vi "GetSetTopSponsorImage.vi"(8 "Which":enum16{"Low", "Mid", "Top"}(ring), 9 "Get/Set":enum16{"Get", "Set"}(ring), 11 "image data":T1) -> (3 "image data out":T1)   [LabVIEW 2013]
uses:
  <vilib>/picture/picture.llb/imagedata.ctl
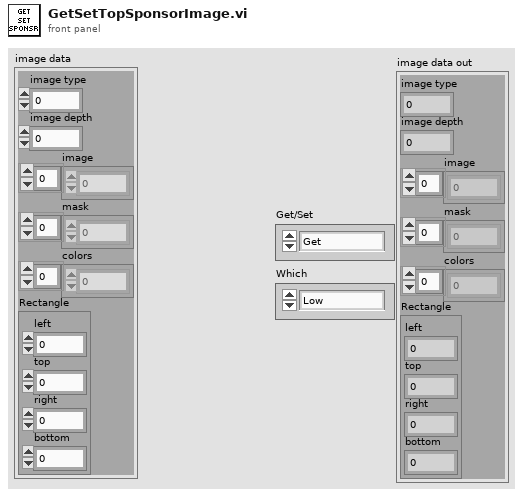
[diagram p1: front panel]
types:
  T1 = typedef "imagedata.ctl" = cluster{"image type":i32, "image depth":i32, "image":u8[], "mask":u8[], "colors":u32[], "Rectangle":cluster{"left":i16, "top":i16, "right":i16, "bottom":i16}}
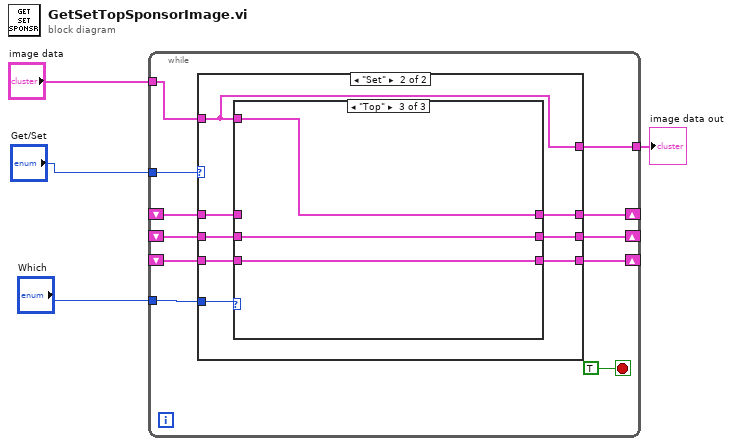
[diagram p0: block diagram]
diagram:
  n1 = while {
    tunnel: "image data" -> [w14]
    shift-right: [w6] -> _
    shift-left: _ -> [w11]
    tunnel: "Get/Set" -> [w15]
    shift-right: [w8] -> _
    shift-left: _ -> [w10]
    shift-right: [w7] -> _
    shift-left: _ -> [w9]
    tunnel: "Which" -> [w12]
    tunnel: [w5] -> w1
    stop <- TRUE stop-if-true
    n2 = case shown="\"Set\"" w15 {
      tunnel: w14 -> [_ w34]
      tunnel: w12 -> [w23 w33]
      tunnel: w11 -> [w22 w40]
      tunnel: w10 -> [w21 w39]
      tunnel: w9 -> [w20 w38]
      tunnel: [w18 w37] -> w8
      tunnel: [w16 w36] -> w7
      tunnel: [w17 w35] -> w6
      tunnel: [w19 w34] -> w5
      frame "Get", Default {
        n3 = case shown="\"Top\"" w23 {
          tunnel: w22 -> [w25 w28 w30]
          tunnel: w21 -> [w26 w29 w32]
          tunnel: w20 -> [w24 w27 w31]
          tunnel: [w24 w29 w30] -> w19
          tunnel: [w26 w29 w32] -> w18
          tunnel: [w25 w28 w30] -> w17
          tunnel: [w24 w27 w31] -> w16
          frame "Low", Default {
          }
          frame "Mid" {
          }
          frame "Top" {
          }
        }
      }
      frame "Set" {
        n4 = case shown="\"Top\"" w33 {
          tunnel: w40 -> [w42 w45 _]
          tunnel: w39 -> [w41 _ w48]
          tunnel: w38 -> [_ w44 w47]
          tunnel: [w41 w46 w48] -> w37
          tunnel: w34 -> [w43 w46 w49]
          tunnel: [w43 w44 w47] -> w36
          tunnel: [w42 w45 w49] -> w35
          frame "Low", Default {
          }
          frame "Mid" {
          }
          frame "Top" {
          }
        }
      }
    }
  }
  "image data out" <- w1
